vi "Self-Sort.vi"(7 "SubComponent List":refnum<class "1553 SubComponent.lvclass">[](array[class]), 8 "error in (no error)":errorcluster, 11 "Bus Controller in":refnum<class "Bus Controller.lvclass">) -> (0 "error out":errorcluster, 5 "SubComponent List out":refnum<class "1553 SubComponent.lvclass">[](array[class]))   [LabVIEW 2016, in "BCI-1553 API.lvlib" / "Bus Controller.lvclass"]
doc: "<DO NOT CALL>\n\nVirtual: All the children who decide to implement this will need to provide a means for locating themselves in the SubComonent List and updating their location appropriately."
uses:
  Bus Controller.lvclass
  1553 SubComponent/1553 SubComponent.lvclass
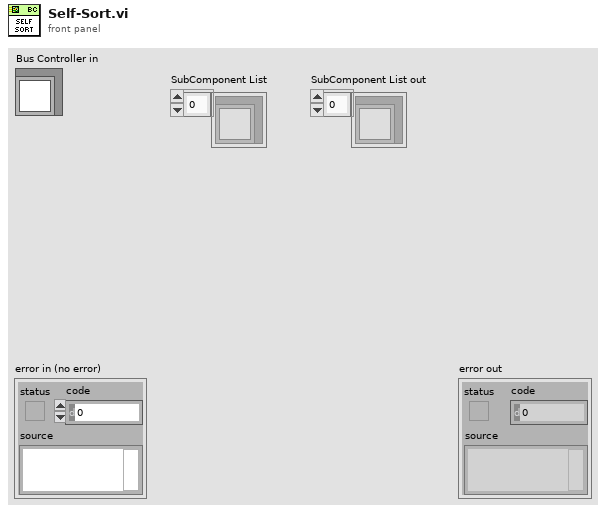
[diagram p1: front panel]
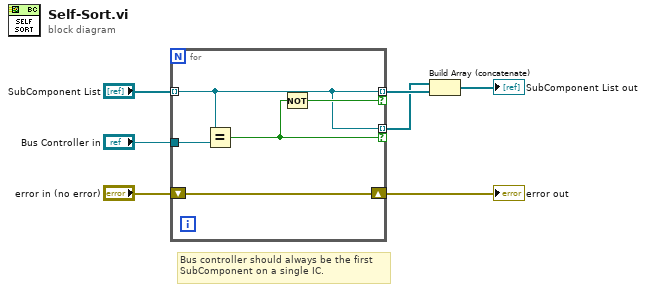
[diagram p0: block diagram]
diagram:
  # "Bus controller should always be the first\nSubComponent on a single IC."
  n1 = for {
    shift-right: [w12] -> w4
    shift-left: "error in (no error)" -> [w12]
    tunnel: "Bus Controller in" -> [w11]
    tunnel: "SubComponent List" -> [w9] mode=indexing
    tunnel: [w9] -> w7 mode=indexing if=w10
    tunnel: [w9] -> w6 mode=indexing if=w8
    n2 = Equal?(x=w9, y=w11) -> (x = y?=w8:bool)
    n3 = Not(x=w8) -> (.not. x?=w10:bool)
  }
  "error out" <- w4
  n4 = Build Array (concatenate)(w6, w7) -> (→"SubComponent List out":refnum<class "1553 SubComponent.lvclass">[])
